vi "MotorInterfaceV3.vi"() -> ()   [LabVIEW 2020]
uses:
  <vilib>/DAQmx/create/channels.llb/DAQmx Create Channel (CO-Pulse Generation-Frequency).vi
  <vilib>/DAQmx/configure/timing.llb/DAQmx Timing (Sample Clock).vi
panel:
  in  "frequency":dbl=10.0 format="%0.2p"
  out "Fault":bool
  out "Direction Test\nPort 0_2":bool[](array[boolean])
  out "Reset Test\nPort 0_1":bool[](array[boolean])
  out "Enable Test\nPort 0_0":bool[](array[boolean])
  in  "Direction":bool
  in  "Reset":bool
  in  "Enable":bool
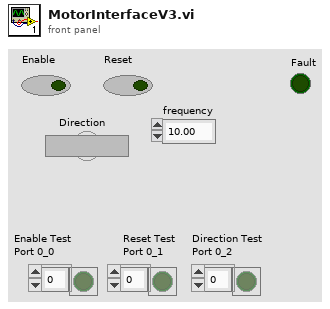
[diagram p1: front panel]
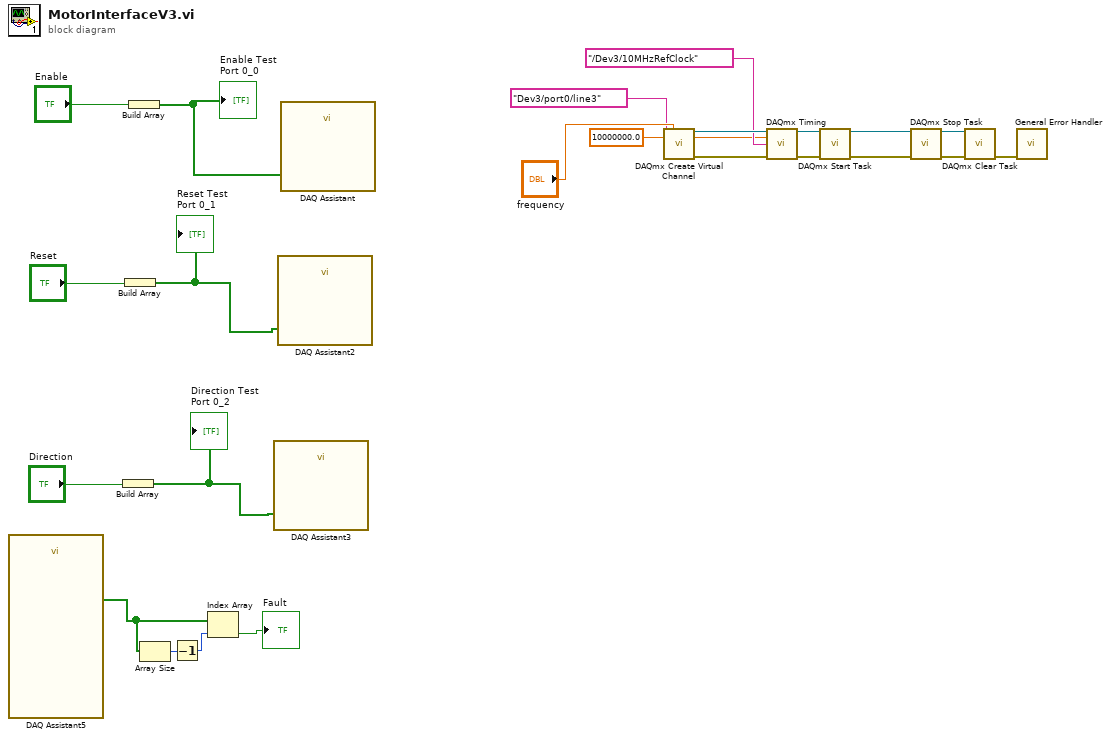
[diagram p0: block diagram]
diagram:
  n1 = call "DAQ Assistant5"() -> ("data"=w16:bool[])  [unwired: 17 in, 2 out]
  n2 = Build Array("Direction") -> (w18:bool[])
  "Direction Test\nPort 0_2" <- w18
  n3 = Build Array("Reset") -> (w20:bool[])
  "Reset Test\nPort 0_1" <- w20
  n4 = Build Array("Enable") -> (w23:bool[])
  "Enable Test\nPort 0_0" <- w23
  n5 = Array Size(array=w16) -> (size(s)=w15:i32)
  n6 = Decrement(x=w15) -> (x-1=w14:i32)
  n7 = Index Array(array=w16, index=w14) -> (element=→"Fault":bool)
  n8 = call "DAQ Assistant3"("data"=w18) -> ()  [unwired: 17 in, 2 out]
  n9 = call "DAQ Assistant2"("data"=w20) -> ()  [unwired: 17 in, 2 out]
  n10 = call "DAQ Assistant"("data"=w23) -> ()  [unwired: 17 in, 2 out]
  n11 = call-poly <vilib>:"DAQmx Create Virtual Channel.vi"("frequency"="frequency", "counter"=tag "Dev3/port0/line3" ("lines")) -> ("task out"=w13:refnum<k21>, "error out"=w12:errorcluster)  [unwired: 12 in]
  n12 = call-poly <vilib>:"DAQmx Timing.vi"("task/channels in"=w13, "rate"=10000000.0, "source"=tag "/Dev3/10MHzRefClock", "error in"=w12) -> ("task out"=w7:refnum<k21>, "error out"=w6:errorcluster)  [unwired: 10 in]
  n13 = call <vilib>:"DAQmx Start Task.vi"("task/channels in"=w7, "error in"=w6) -> ("task out"=w2:refnum<k21>, "error out"=w3:errorcluster)  [unwired: 12 in]
  n14 = call <vilib>:"DAQmx Stop Task.vi"("task/channels in"=w2, "error in"=w3) -> ("task out"=w11:refnum<k21>, "error out"=w10:errorcluster)  [unwired: 12 in]
  n15 = call <vilib>:"DAQmx Clear Task.vi"("task in"=w11, "error in"=w10) -> ("error out"=w9:errorcluster)  [unwired: 13 in]
  n16 = call <vilib>:"General Error Handler.vi"("error in (no error)"=w9) -> ()  [unwired: 10 in, 5 out]
